vi "Get Next Step.vi"(0 "iProcess Step Model in":refnum<class "iProcess Step Model.lvclass">, 11 "error in (no error)":errorcluster) -> (4 "iProcess Step Model out":refnum<class "iProcess Step Model.lvclass">, 12 "Found":bool, 13 "Complete":bool, 14 "Stop":bool, 15 "error out":errorcluster)   [LabVIEW 2017, in "iProcess Step Model.lvlib" / "iProcess Step Model.lvclass"]
uses:
  iProcess Step Model.lvclass
  iProcess Step Model.lvclass/iProcess Step Model.ctl
panel:
  in  "TestErrorHandle":cluster{"Errorcode":i32}
  in  "TestPREREQ":string
  in  "TestCasesensitive":enum16{"NO", "YES"}(ring)
  in  "SFCEnable":enum16{"EMPTY", "ON", "OFF"}(ring)
  in  "LoopEnable":enum16{"EMPTY", "ON", "OFF"}(ring)
  in  "RunInParallel":bool
  in  "TestErrorHandle":cluster{"Errorcode":i32}
  in  "TestSaveResult":bool
  in  "TestHighLimit":string
  in  "TestLowLimit":string
  in  "TestUnit":string
  in  "TestLimitCheck":string
  in  "TestErrorCode":string
  in  "TestPlanName":string
  in  "TestPlan":T1={"TestIndex"=0, "TestProperty"=[], "TestInputParameter"="", "TestRetry"=0, "TestEnable"=FALSE, "TestVIName"="", "TestName"="", "NextStepHandle"={"NextIndex"=0, "TestGotoCounter"=0, "TestNextStep"=enum."If…else", "TestNextViName"=""}}
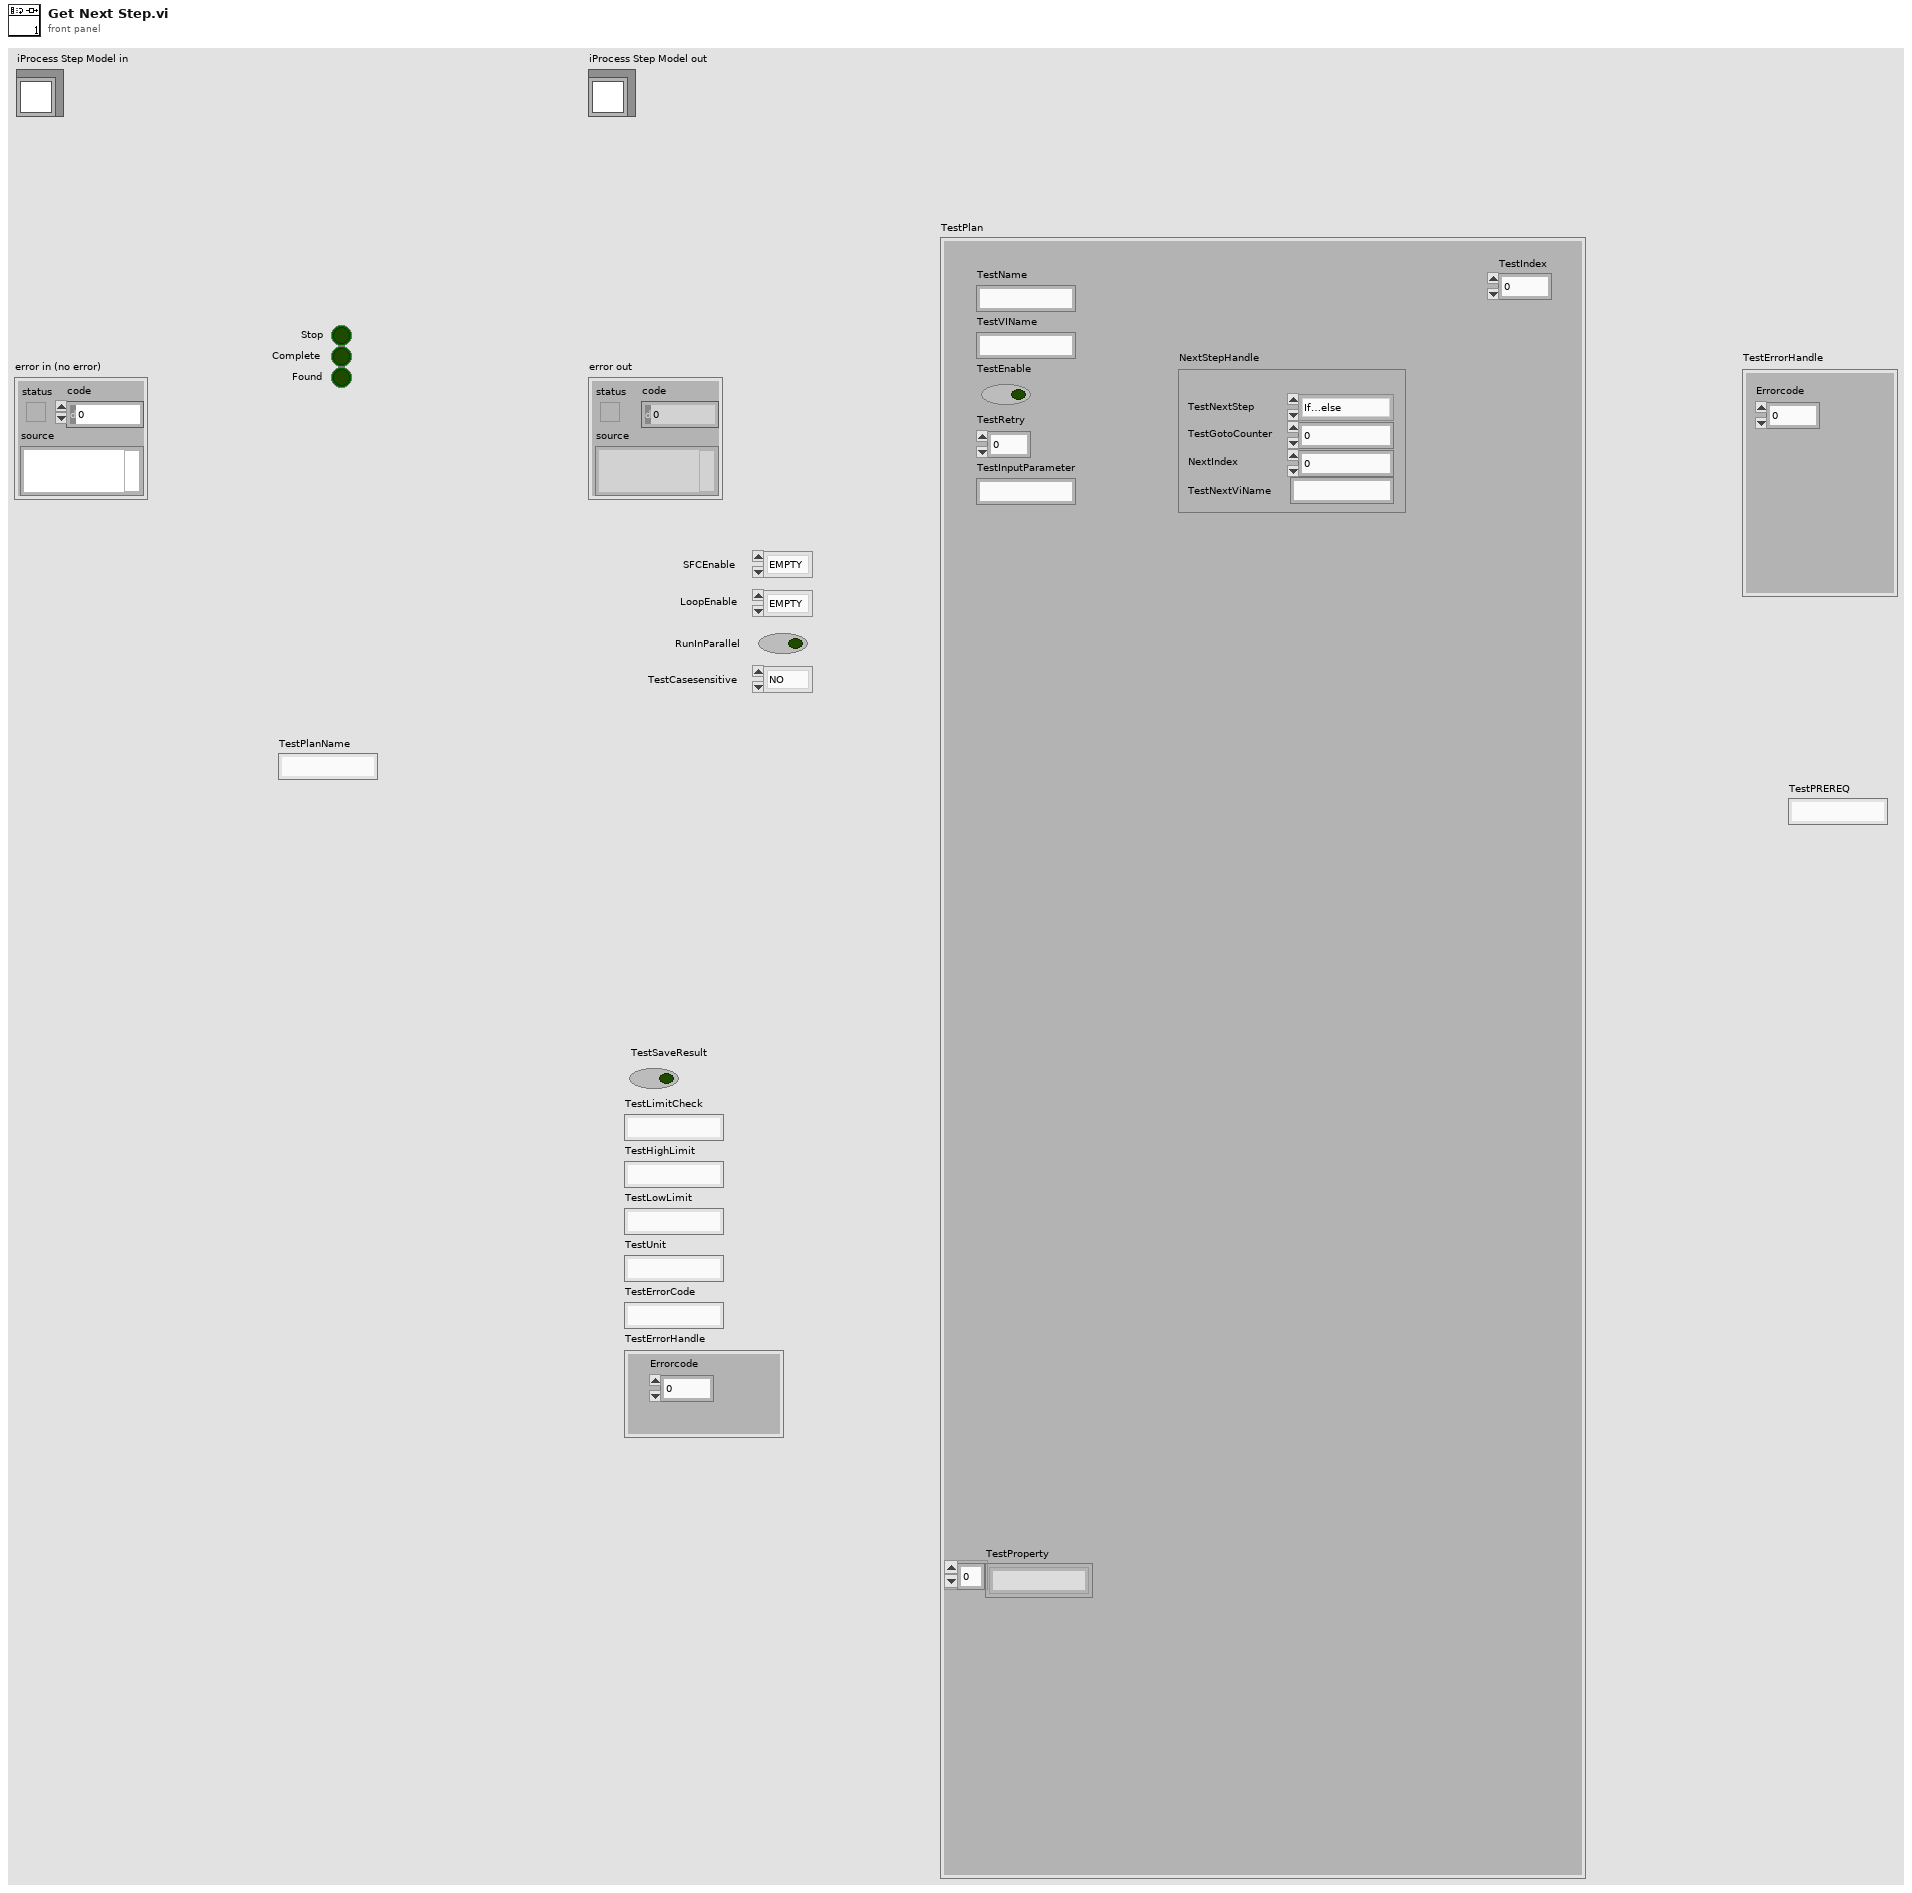
[diagram p1: front panel]
types:
  T1 = cluster{"TestIndex":u64, "TestProperty":string[], "TestInputParameter":string, "TestRetry":u64, "TestEnable":bool, "TestVIName":string, "TestName":string, "NextStepHandle":cluster{"NextIndex":i32, "TestGotoCounter":u64, "TestNextStep":enum16{"None", "Next", "Stop if Fail", "If Fail goto", "Goto", "If Pass goto", "Force Pass", "Force Fail", "If…else", "Switch...case", "Stop Slot", "Pause Slot", "Continue Slot"}, "TestNextViName":string}}
  T2 = cluster{"TestName":string[], "TestVIName":string[], "TestEnable":bool[], "TestRetry":u64[], "TestNextStep":enum16{"None", "Next", "Stop if Fail", "If Fail goto", "Goto", "If Pass goto", "Force Pass", "Force Fail", "If…else", "Switch...case", "Stop Slot", "Pause Slot", "Continue Slot"}[], "TestPREREQ":string[], "TestSaveResult":bool[], "TestInputParameter":string[], "TestHighLimit":string[], "TestLowLimit":string[], "TestIndex":u64[], "TestNextViName":string[], "TestGotoCounter":u64[], "TestUnit":string[], "TestPlanName":string, "ShowResultArray":cluster{"Lenght":i32, "TestNextStep":enum16{"None", "Next", "Stop if Fail", "If Fail goto", "Goto", "If Pass goto", "Force Pass", "Force Fail", "If…else"}[], "TestSaveResult":bool[], "ErrorCode":string[], "LimitCheck":string[]}[], "StartIndex":i32[], "TestErrorHandle":string[], "TestLimitCheck":string[], "TestProperty":string[], "TestCasesensitive":enum16{"NO", "YES"}[], "TestErrorCode":string[], "SFCEnable":enum16{"EMPTY", "ON", "OFF"}[], "LoopEnable":enum16{"EMPTY", "ON", "OFF"}[], "RunInParallel":bool[]}[]
  T3 = cluster{"TestName":string[], "TestVIName":string[], "TestEnable":bool[], "TestRetry":u64[], "TestNextStep":enum16{"None", "Next", "Stop if Fail", "If Fail goto", "Goto", "If Pass goto", "Force Pass", "Force Fail", "If…else", "Switch...case", "Stop Slot", "Pause Slot", "Continue Slot"}[], "TestPREREQ":string[], "TestSaveResult":bool[], "TestInputParameter":string[], "TestHighLimit":string[], "TestLowLimit":string[], "TestIndex":u64[], "TestNextViName":string[], "TestGotoCounter":u64[], "TestUnit":string[], "TestPlanName":string, "ShowResultArray":cluster{"Lenght":i32, "TestNextStep":enum16{"None", "Next", "Stop if Fail", "If Fail goto", "Goto", "If Pass goto", "Force Pass", "Force Fail", "If…else"}[], "TestSaveResult":bool[], "ErrorCode":string[], "LimitCheck":string[]}[], "StartIndex":i32[], "TestErrorHandle":string[], "TestLimitCheck":string[], "TestProperty":string[], "TestCasesensitive":enum16{"NO", "YES"}[], "TestErrorCode":string[], "SFCEnable":enum16{"EMPTY", "ON", "OFF"}[], "LoopEnable":enum16{"EMPTY", "ON", "OFF"}[], "RunInParallel":bool[]}
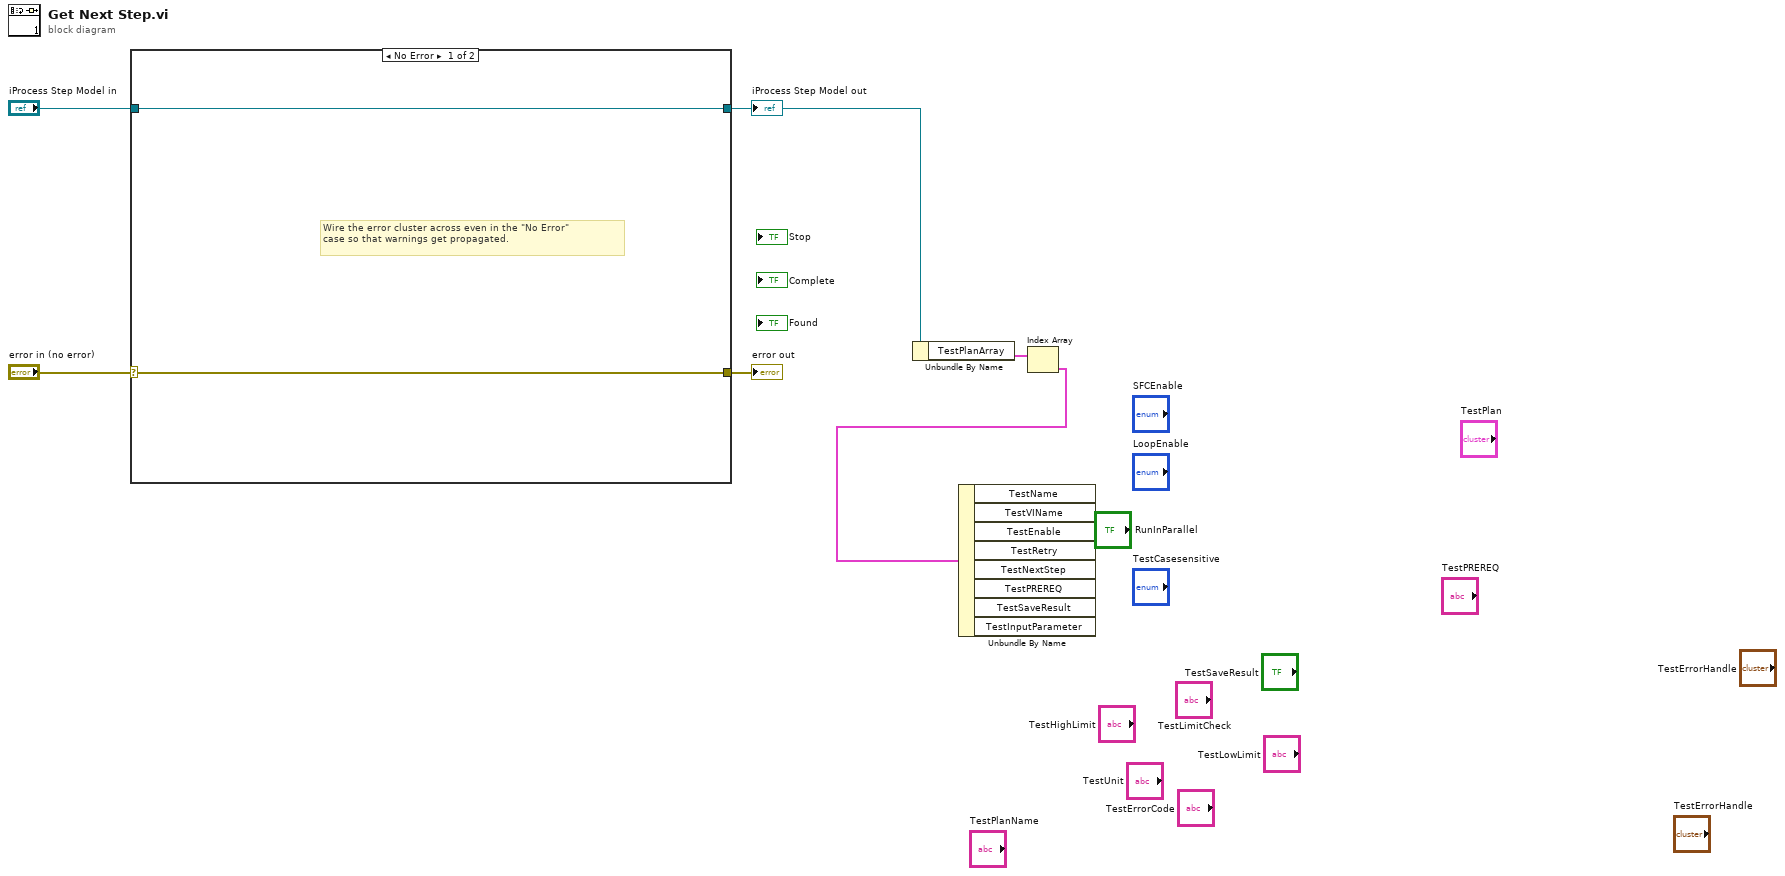
[diagram p0: block diagram]
diagram:
  n1 = case shown="No Error" "error in (no error)" {
    selector: "error in (no error)" -> [w7 w10]
    tunnel: [w7 w10] -> w5
    tunnel: [w8 w9] -> w3
    tunnel: "iProcess Step Model in" -> [w8 w9]
    frame No Error {
      # "Wire the error cluster across even in the \"No Error\"\ncase so that warnings get propagated."
    }
    frame Error {
    }
  }
  "error out" <- w5
  "iProcess Step Model out" <- w3
  n2 = Unbundle By Name(w3) -> ("TestPlanArray"=w2:T2)
  n3 = Index Array(array=w2) -> (element=w1:T3)  [unwired: 1 in]
  n4 = Unbundle By Name(w1) -> ()  [unwired: 8 out]
